vi "路径转换.vi"(1 "input path":path) -> (0 "output path":path)   [LabVIEW 2014]
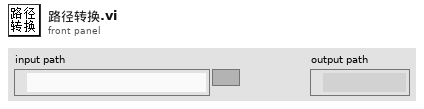
[diagram p1: front panel]
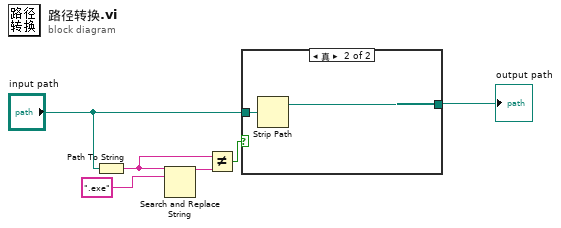
[diagram p0: block diagram]
diagram:
  n1 = Path To String(path="input path") -> (string=w2:string)
  n2 = Search and Replace String(input string=w2, search string=".exe" ("搜索字符串")) -> (result string=w3:string)  [unwired: 6 in, 3 out]
  n3 = Not Equal?(x=w2, y=w3) -> (x != y?=w1:bool)
  n4 = case shown="真" w1 {
    tunnel: [w7 w8] -> w6
    tunnel: "input path" -> [w7 w9]
    frame False {
    }
    frame True {
      n5 = Strip Path(path=w9) -> (stripped path=w8:path)  [unwired: 1 out]
    }
  }
  "output path" <- w6
